vi "E2A_Waveform.vi"(11 "Data in":dbl[](array[numeric])) -> (3 "WF out":waveform(dbl)[](array[waveform]))   [LabVIEW 2022 SP3]
panel:
  out "appended array":dbl[](array[numeric])
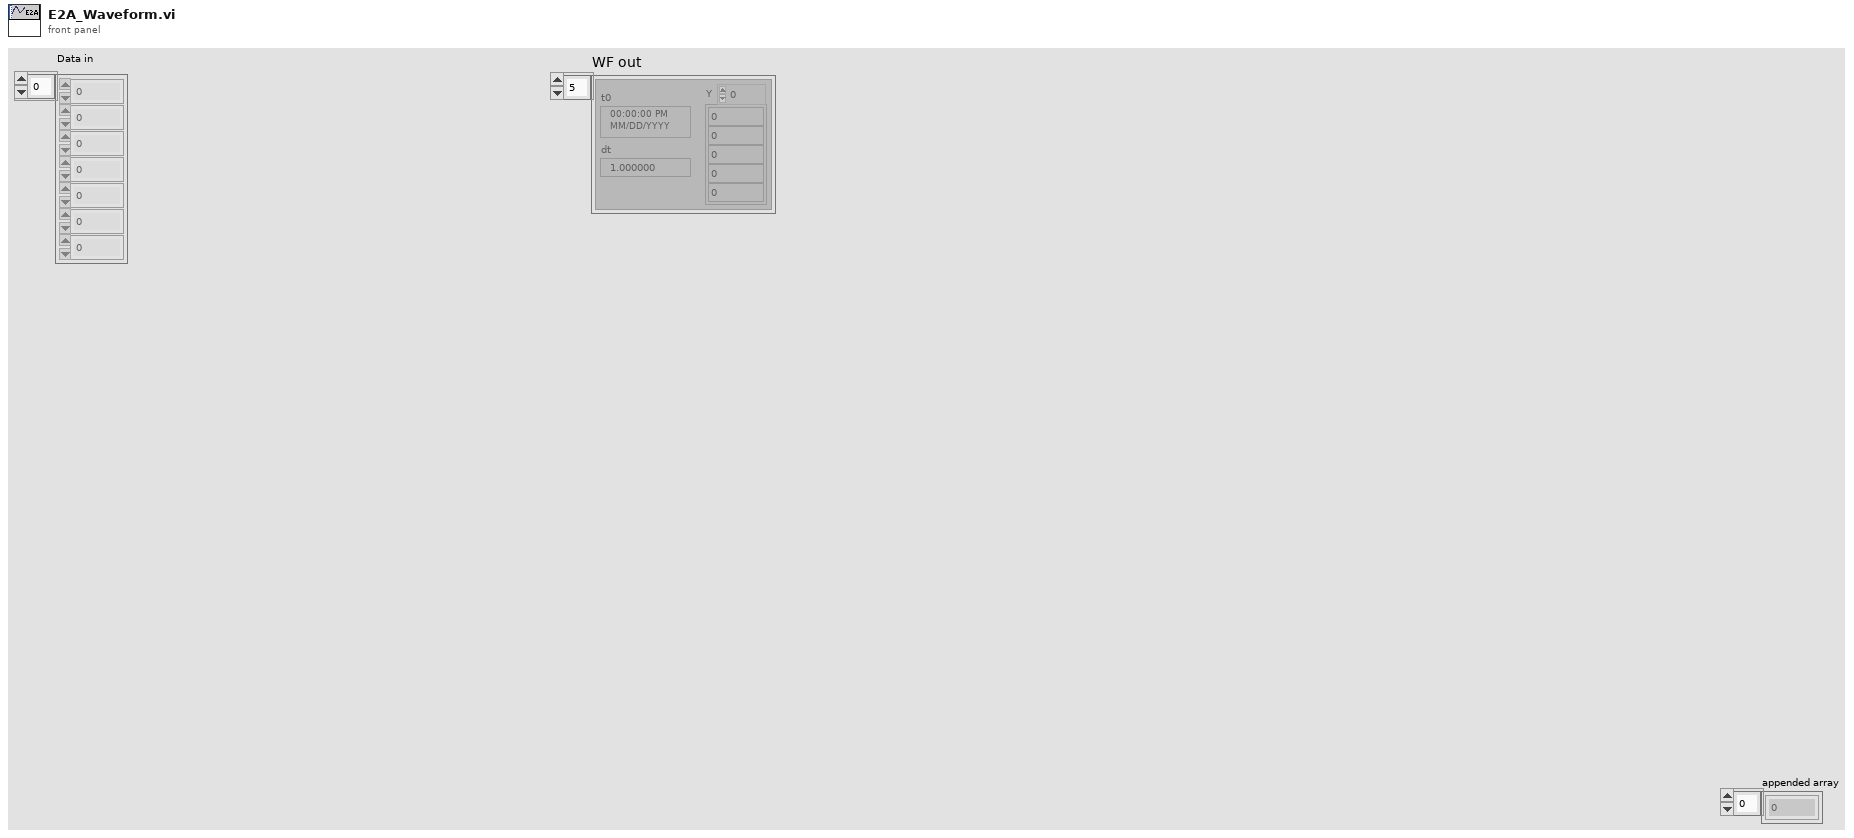
[diagram p1: front panel]
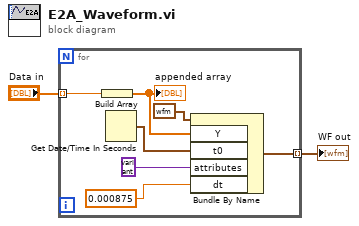
[diagram p0: block diagram]
diagram:
  n1 = for {
    tunnel: "Data in" -> [w6] mode=indexing
    tunnel: [w8] -> w2 mode=indexing
    n2 = Build Array(w6) -> (w5:dbl[])
    "appended array" <- w5
    n3 = Get Date/Time In Seconds() -> (seconds since 1Jan1904=w4:timestamp)
    n4 = Bundle By Name(cluster=waveform(dbl) {"t0"=timestamp(0 s since 1904-01-01), "dt"=1.0, "Y"=[]} ("waveform"), "Y"=w5, "t0"=w4, "attributes"=variant, "dt"=0.000875) -> (w8:waveform(dbl))
  }
  "WF out" <- w2
